vi "Queue Comms Flush Enqueue.vi"(8 "error in (no error)":errorcluster, 11 "element":T1) -> (0 "error out":errorcluster)   [LabVIEW 2018, in "Vibration.lvlib"]
doc: "This subVI flushes the queue then enqueues an element in to the communications queue to be handleds"
uses:
  Vibration.lvlib
  Private Controls/Module Data.ctl
  Private Controls/Module Action.ctl
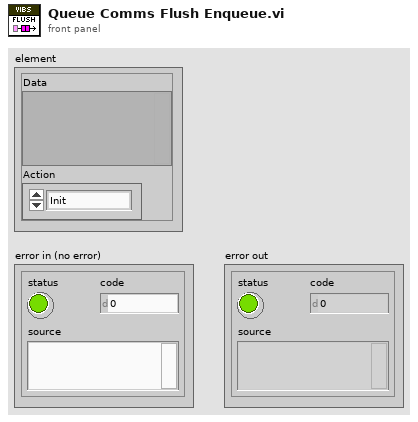
[diagram p1: front panel]
types:
  T1 = typedef "Vibration.lvlib/Module Data.ctl" = cluster{"Data":variant, "Action":T2}
  T2 = typedef "Vibration.lvlib/Module Action.ctl" = enum16{"Init", "Error"}
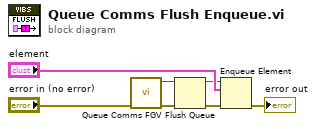
[diagram p0: block diagram]
diagram:
  n1 = call "Queue Comms FGV.vi"("error in (no error)"="error in (no error)") -> ("error out"=w4:errorcluster, "Queue out"=w3:refnum<queue>)  [unwired: 9 in]
  n2 = Flush Queue(queue=w3, error in (no error)=w4) -> (queue out=w2:refnum<queue>, error out=w1:errorcluster)  [unwired: 1 out]
  n3 = Enqueue Element(queue=w2, element="element", error in (no error)=w1) -> (error out=→"error out":errorcluster)  [unwired: 1 in, 2 out]
